vi "Listbox - Initialize Test.vi"(8 "error in (no error)":errorcluster, 11 "SV B-M In":refnum<class "SV B-M (Host).lvclass">) -> (0 "error out":errorcluster, 3 "SV B-M Out":refnum<class "SV B-M (Host).lvclass">)   [LabVIEW 2015, in "SV B-M (Host).lvclass"]
doc: "Initializes the listbox for a new individual test within a sequence."
uses:
  SV B-M (Host).lvclass
  SV B-M (Host).lvclass/SV B-M (Host).ctl
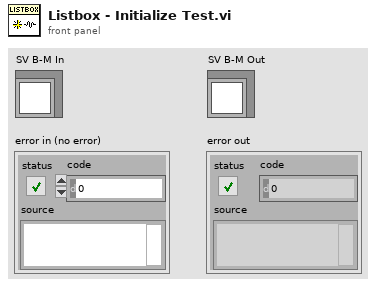
[diagram p1: front panel]
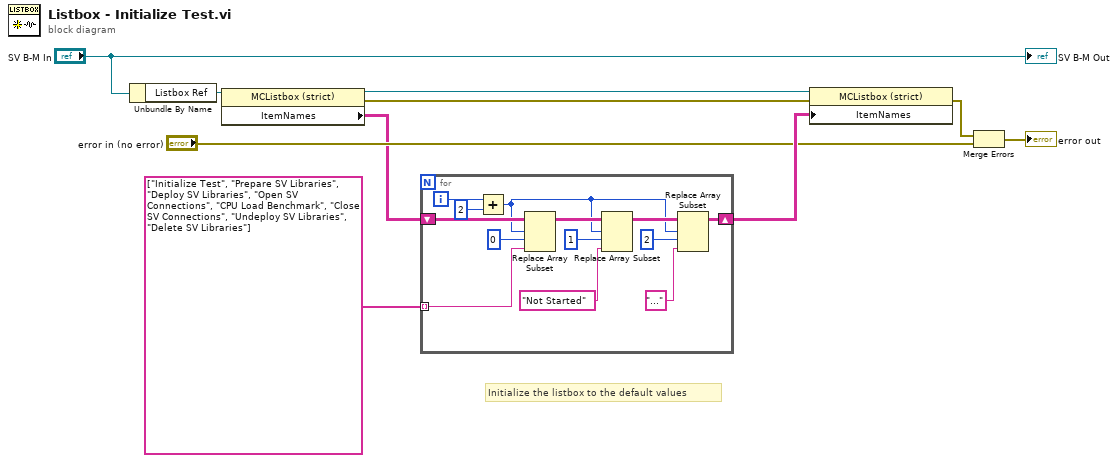
[diagram p0: block diagram]
diagram:
  # "Initialize the listbox to the default values"
  n1 = Unbundle By Name("SV B-M In") -> ("Listbox Ref"=w1:refnum<vi>)
  n2 = property class="MCListbox (strict)"(reference=w1) -> (reference out=w5:refnum<vi>, error out=w4:errorcluster, "ItemNames"=w3:string[][])  [unwired: 1 in]
  n3 = for {
    shift-right: [w17] -> w10
    shift-left: w3 -> [w23]
    tunnel: string[] ["Initialize Test", "Prepare SV Libraries", "Deploy SV Libraries", "Open SV Connections", "CPU Load Benchmark", "Close SV Connections", "Undeploy SV Libraries", "Delete SV Libraries"] -> [w14] mode=indexing
    i -> [w13]
    n4 = Add(x=w13, y=2) -> (x+y=w12:i32)
    n5 = Replace Array Subset(array=w23, new element=w14, index (row)=w12, index (col)=0 ("disabled index (col)")) -> (w20:string[][])
    n6 = Replace Array Subset(array=w20, new element="Not Started", index (row)=w12, index (col)=1 ("disabled index (col)")) -> (w18:string[][])
    n7 = Replace Array Subset(array=w18, new element="...", index (row)=w12, index (col)=2 ("disabled index (col)")) -> (w17:string[][])
  }
  n8 = property class="MCListbox (strict)"(reference=w5, error in=w4, "ItemNames"=w10) -> (error out=w7:errorcluster)  [unwired: 1 out]
  n9 = Merge Errors(w7, "error in (no error)") -> (→"error out":errorcluster)
  "SV B-M Out" <- "SV B-M In"
